vi "Read_From_CSV_CFR_CWB.vi"(8 "time delay (s)":dbl=60.0, 9 "input string":string, 10 "Spreadsheet path (.csv)":path=path "C:/Users/husmith/Desktop/MyData.csv") -> (2 "output data":string[](array[string]), 3 "time stamp":timestamp)   [LabVIEW 2014]
uses:
  <vilib>/Utility/file.llb/Read From Spreadsheet File (string).vi
panel:
  out "Timestamp array (s)":dbl[](array[numeric]) format="%#_11g"
  out "last element of Timestamp array (s)":dbl format="%#_10g"
  out "Timestamp of last element of Timestamp array (s)":timestamp
  out "Input Timestamp (s)":dbl format="%#_10g"
  out "Input Timestamp":timestamp
  out "closest element":dbl format="%#_11g"
  out "closest index":i32
  out "Data array":string[][](array[string])
  out "Timestamp array":string[][](array[string])
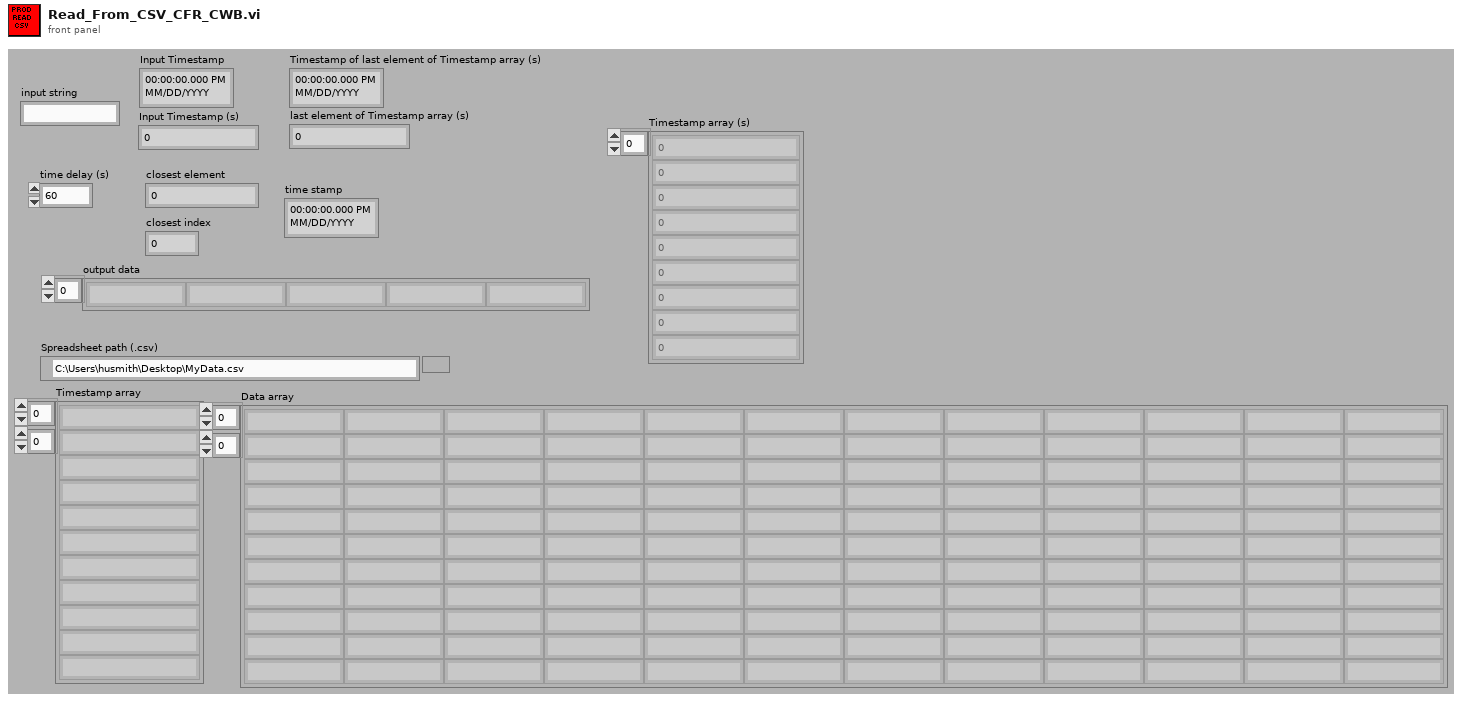
[diagram p1: front panel]
types:
  T1 = cluster{"second":i32, "minute":i32, "hour":i32, "day of month":i32, "month":i32, "year":i32, "day of week":i32, "day of year":i32, "is DST":i32}
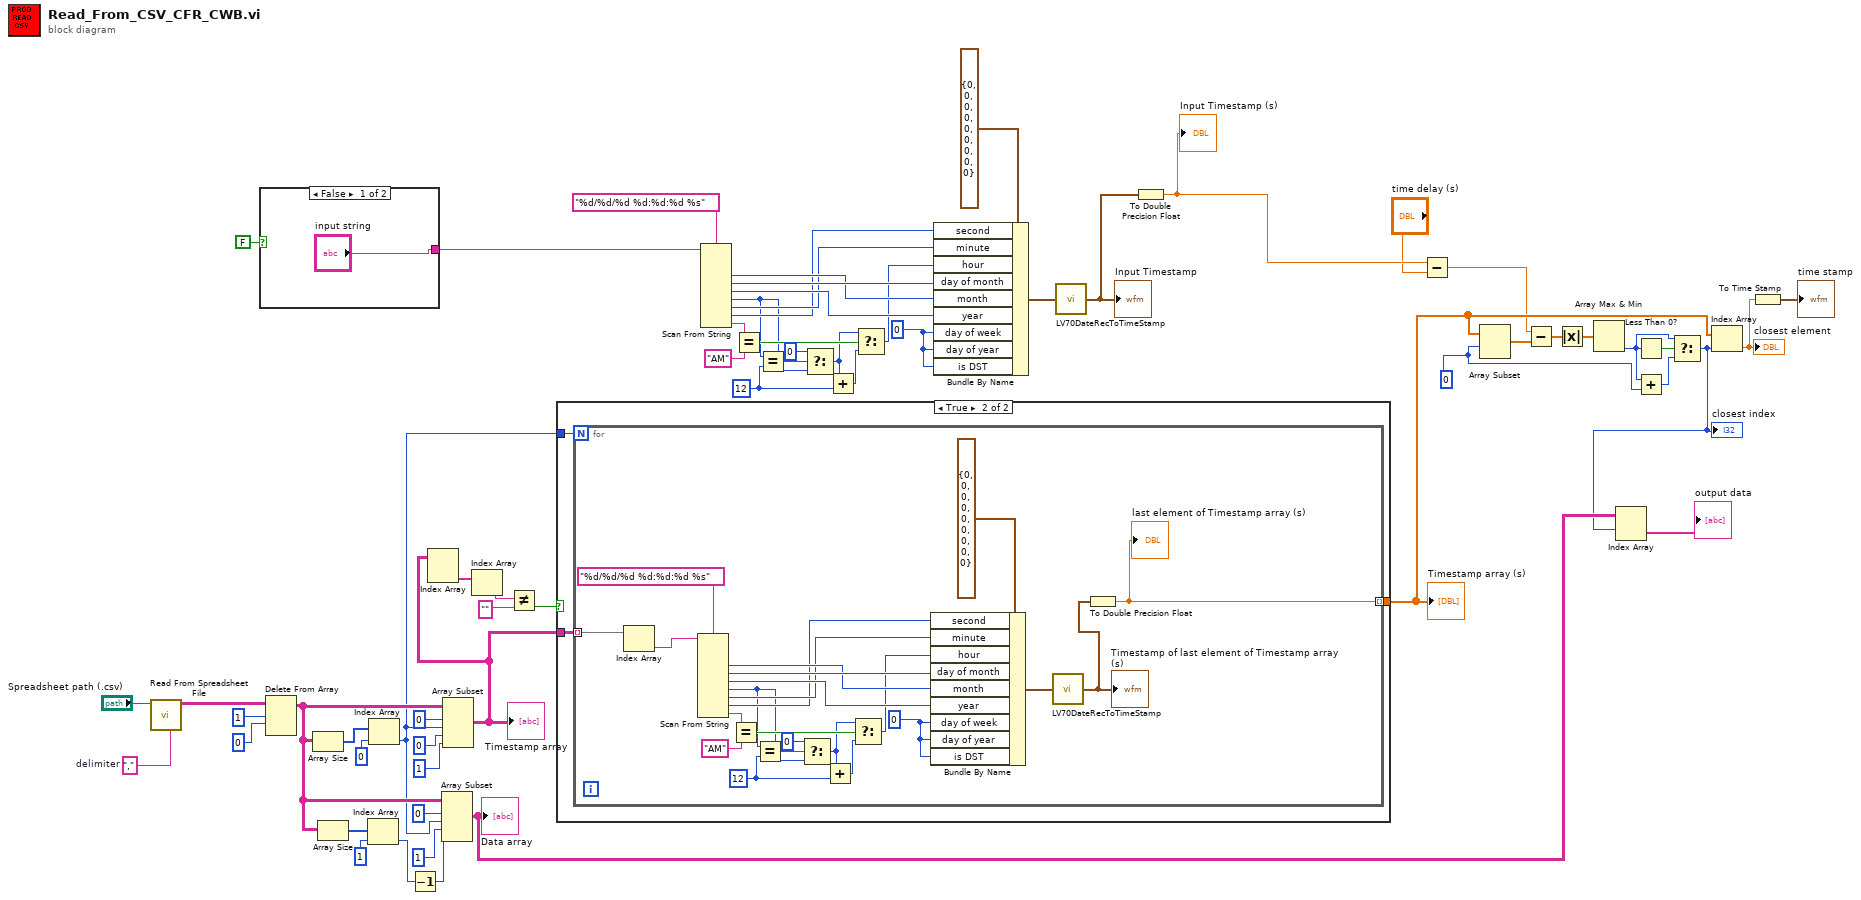
[diagram p0: block diagram]
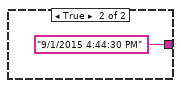
[diagram p2: hidden frame]
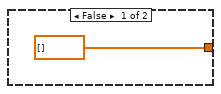
[diagram p3: hidden frame]
diagram:
  w23 = 12 ("y")
  w34 = 0
  w38 = 0 ("start index (0)")
  w60 = ","  # delimiter
  n1 = call-poly <vilib>:"Read From Spreadsheet File.vi"("delimiter (\\t)"=w60, "file path (dialog if empty)"="Spreadsheet path (.csv)") -> ("all rows"=w59:string[][])  [unwired: 5 in, 4 out]
  n2 = case shown="False" FALSE {
    tunnel: ["input string" "9/1/2015 4:44:30 PM"] -> w18
    frame False {
    }
    frame True {
    }
  }
  n3 = Delete From Array(array=w59, length=1, index (row)=0) -> (array with subset deleted=w48:string[][])  [unwired: 1 in, 1 out]
  n4 = Array Size(array=w48) -> (size(s)=w53:i32[])
  n5 = Array Size(array=w48) -> (size(s)=w47:i32[])
  n6 = Index Array(array=w47, index=1) -> (element=w46:i32)
  n7 = Index Array(array=w53, index=0) -> (element=w16:i32)
  n8 = Decrement(x=w46) -> (x-1=w45:i32)
  n9 = Array Subset(array=w48, index (row)=0 ("index"), length (row)=w16, index (col)=1 ("index"), length (col)=w45) -> (w4:string[][])
  "Data array" <- w4
  n10 = Array Subset(array=w48, index (row)=0 ("index"), length (row)=w16, index (col)=0 ("index"), length (col)=1 ("length")) -> (w8:string[][])
  "Timestamp array" <- w8
  n11 = Index Array(array=w8) -> (element=w7:string[])  [unwired: 2 in]
  n12 = Index Array(array=w7) -> (element=w6:string)  [unwired: 1 in]
  n13 = Not Equal?(x=w6, y="") -> (x != y?=w9:bool)
  n14 = case shown="True" w9 {
    tunnel: w16 -> [_ w67]
    tunnel: w8 -> [_ w66]
    tunnel: [dbl[] [] w65] -> w15
    frame False {
    }
    frame True {
      n15 = for {
        N: w67 -> [_]
        tunnel: [w70] -> w65 mode=indexing
        tunnel: w66 -> [w69] mode=indexing
        w76 = 12 ("y")
        w87 = 0
        n16 = Index Array(array=w69) -> (element=w68:string)  [unwired: 1 in]
        n17 = Scan From String "Scan From String"(format string="%d/%d/%d %d:%d:%d %s", input string=w68) -> (output 1=w85:i32, output 2=w86:i32, output 3=w84:i32, output 4=w74:i32, output 5=w83:i32, output 6=w82:i32, output 7=w81:string)  [unwired: 9 in, 3 out]
        n18 = Equal?(x=w81, y="AM") -> (x = y?=w77:bool)
        n19 = Equal?(x=w74, y=w76) -> (x = y?=w75:bool)
        n20 = Select(t=0, s=w75, f=w74) -> (s? t:f=w73:i32)
        n21 = Add(x=w73, y=w76) -> (x+y=w78:i32)
        n22 = Select(t=w73, s=w77, f=w78) -> (s? t:f=w79:i32)
        n23 = Bundle By Name(cluster=T1 {"second"=0, "minute"=0, "hour"=0, "day of month"=0, "month"=0, "year"=0, "day of week"=0, "day of year"=0, "is DST"=0} ("date time rec"), "second"=w82, "minute"=w83, "hour"=w79, "day of month"=w86, "month"=w85, "year"=w84, "day of week"=w87, "day of year"=w87, "is DST"=w87) -> (w88:T1)
        n24 = call <vilib>:"LV70DateRecToTimeStamp.vi"("date time rec"=w88) -> ("Time Stamp"=w71:timestamp)
        "Timestamp of last element of Timestamp array (s)" <- w71
        n25 = To Double Precision Float(number=w71) -> (double precision float=w70:dbl)
        "last element of Timestamp array (s)" <- w70
      }
    }
  }
  "Timestamp array (s)" <- w15
  n26 = Scan From String "Scan From String"(format string="%d/%d/%d %d:%d:%d %s", input string=w18) -> (output 1=w32:i32, output 2=w33:i32, output 3=w31:i32, output 4=w21:i32, output 5=w30:i32, output 6=w29:i32, output 7=w28:string)  [unwired: 9 in, 3 out]
  n27 = Equal?(x=w28, y="AM") -> (x = y?=w24:bool)
  n28 = Equal?(x=w21, y=w23) -> (x = y?=w22:bool)
  n29 = Select(t=0, s=w22, f=w21) -> (s? t:f=w20:i32)
  n30 = Add(x=w20, y=w23) -> (x+y=w25:i32)
  n31 = Select(t=w20, s=w24, f=w25) -> (s? t:f=w26:i32)
  n32 = Bundle By Name(cluster=T1 {"second"=0, "minute"=0, "hour"=0, "day of month"=0, "month"=0, "year"=0, "day of week"=0, "day of year"=0, "is DST"=0} ("date time rec"), "second"=w29, "minute"=w30, "hour"=w26, "day of month"=w33, "month"=w32, "year"=w31, "day of week"=w34, "day of year"=w34, "is DST"=w34) -> (w35:T1)
  n33 = call <vilib>:"LV70DateRecToTimeStamp.vi"("date time rec"=w35) -> ("Time Stamp"=w17:timestamp)
  "Input Timestamp" <- w17
  n34 = To Double Precision Float(number=w17) -> (double precision float=w14:dbl)
  "Input Timestamp (s)" <- w14
  n35 = Subtract(x=w14, y="time delay (s)") -> (x-y=w13:dbl)
  n36 = Array Subset(array=w15, index=w38) -> (w39:dbl[])  [unwired: 1 in]
  n37 = Subtract(x=w13, y=w39) -> (x-y=w44:dbl[])
  n38 = Absolute Value(x=w44) -> (abs(x)=w43:dbl[])
  n39 = Array Max & Min(array=w43) -> (min index (indices)=w41:i32)  [unwired: 3 out]
  n40 = Less Than 0?(x=w41) -> (x < 0?=w42:bool)
  n41 = Add(x=w41, y=w38) -> (x+y=w40:i32)
  n42 = Select(t=w41, s=w42, f=w40) -> (s? t:f=w3:i32)
  "closest index" <- w3
  n43 = Index Array(array=w4, index (row)=w3) -> (element=→"output data":string[])  [unwired: 1 in]
  n44 = Index Array(array=w15, index=w3) -> (element=w12:dbl)
  "closest element" <- w12
  n45 = To Time Stamp(1:w12) -> (0:→"time stamp":timestamp)
